vi "MV set power.vi"(8 "error in (no error)":errorcluster, 10 "power (W)":dbl=0.2 min=0.2 max=5.0 step=0.01 format="%.2g", 11 "VISA resource name":refnum<visa-resource-name>) -> (0 "error out":errorcluster, 3 "VISA resource name out":refnum<visa-resource-name>)   [LabVIEW 2023, in "Millennia V.lvclass"]
doc: "Sets the power of the Millennia V laser."
uses:
  Millennia V.lvclass
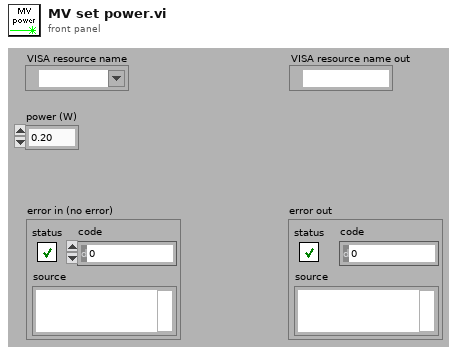
[diagram p1: front panel]
types:
  T1 = enum16{"read only", "write only", "write + read"}
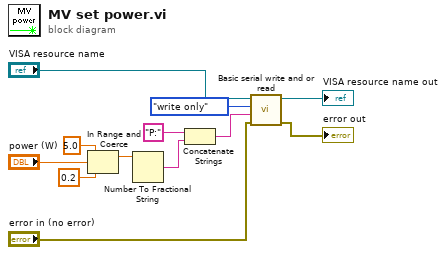
[diagram p0: block diagram]
diagram:
  n1 = In Range and Coerce(upper limit=5.0, x="power (W)", lower limit=0.2) -> (coerced(x)=w7:dbl)  [unwired: 1 out]
  n2 = Number To Fractional String(number=w7) -> (F-format string=w5:string)  [unwired: 3 in]
  n3 = Concatenate Strings("P:" ("write string"), w5) -> (w4:string)
  n4 = call "Basic serial write and or read.vi"("error in (no error)"="error in (no error)", "write string"=w4, "action"=T1."write only", "VISA resource name"="VISA resource name") -> ("error out"=→"error out":errorcluster, "VISA resource name out"=→"VISA resource name out":refnum<visa-resource-name>)  [unwired: 4 in, 2 out]
